vi "DownsampleStage3_5761_10MHzPID.vi"(8 "valid in":bool, 9 "reset":bool, 11 "Data in":fxp<+/-,32,14>[](array[numeric])=[0.0, 0.0, 0.0, 0.0, 0.0, 0.0, 0.0, 0.0]) -> (0 "valid out":bool, 3 "data out":fxp<+/-,32,14>[](array[numeric]))   [LabVIEW 2018]
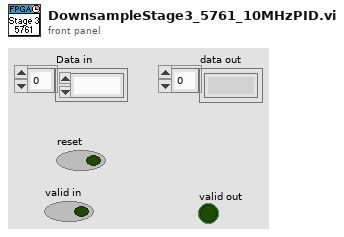
[diagram p1: front panel]
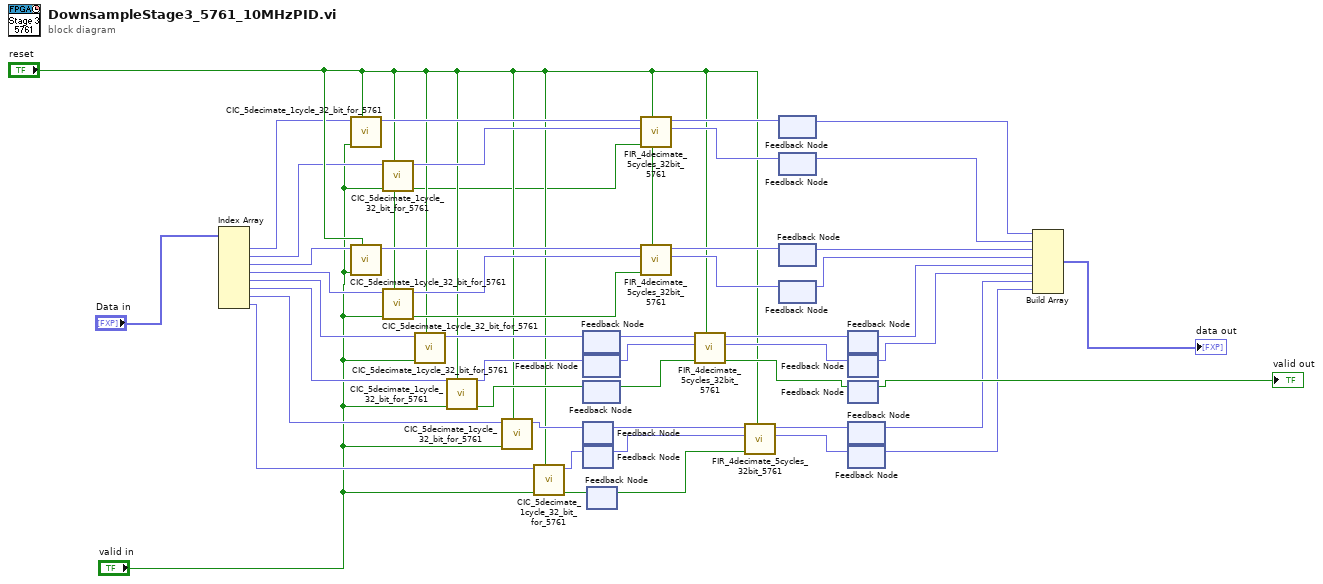
[diagram p0: block diagram]
diagram:
  n1 = Index Array(array="Data in") -> (element #1=w6:fxp<+/-,32,14>, element #2=w5:fxp<+/-,32,14>, element #3=w46:fxp<+/-,32,14>, element #4=w44:fxp<+/-,32,14>, element #5=w43:fxp<+/-,32,14>, element #6=w42:fxp<+/-,32,14>, element #7=w23:fxp<+/-,32,14>, element #8=w22:fxp<+/-,32,14>)  [unwired: 8 in]
  n2 = call "CIC_5decimate_1cycle_32_bit_for_5761.vi"("reset"="reset", "valid in"="valid in", "Data in"=w6) -> ("Data out"=w8:fxp<+/-,32,14>)  [unwired: 7 in, 1 out]
  n3 = call "CIC_5decimate_1cycle_32_bit_for_5761.vi"("reset"="reset", "valid in"="valid in", "Data in"=w46) -> ("Data out"=w35:fxp<+/-,32,14>)  [unwired: 7 in, 1 out]
  n4 = call "CIC_5decimate_1cycle_32_bit_for_5761.vi"("reset"="reset", "valid in"="valid in", "Data in"=w5) -> ("valid out"=w4:bool, "Data out"=w9:fxp<+/-,32,14>)  [unwired: 7 in]
  n5 = call "CIC_5decimate_1cycle_32_bit_for_5761.vi"("reset"="reset", "valid in"="valid in", "Data in"=w44) -> ("valid out"=w33:bool, "Data out"=w34:fxp<+/-,32,14>)  [unwired: 7 in]
  n6 = call "CIC_5decimate_1cycle_32_bit_for_5761.vi"("reset"="reset", "valid in"="valid in", "Data in"=w43) -> ("Data out"=w41:fxp<+/-,32,14>)  [unwired: 7 in, 1 out]
  n7 = call "CIC_5decimate_1cycle_32_bit_for_5761.vi"("reset"="reset", "valid in"="valid in", "Data in"=w42) -> ("valid out"=w39:bool, "Data out"=w40:fxp<+/-,32,14>)  [unwired: 7 in]
  n8 = call "CIC_5decimate_1cycle_32_bit_for_5761.vi"("reset"="reset", "valid in"="valid in", "Data in"=w23) -> ("Data out"=w17:fxp<+/-,32,14>)  [unwired: 7 in, 1 out]
  n9 = call "CIC_5decimate_1cycle_32_bit_for_5761.vi"("reset"="reset", "valid in"="valid in", "Data in"=w22) -> ("valid out"=w13:bool, "Data out"=w16:fxp<+/-,32,14>)  [unwired: 7 in]
  n10 = feedback #1() -> (w38:fxp<+/-,32,14>)  [unwired: 1 in]
  n11 = feedback-in #1(w41) -> ()
  n12 = feedback #2() -> (w37:fxp<+/-,32,14>)  [unwired: 1 in]
  n13 = feedback-in #2(w40) -> ()
  n14 = feedback #3() -> (w36:bool)  [unwired: 1 in]
  n15 = feedback-in #3(w39) -> ()
  n16 = feedback #4() -> (w18:fxp<+/-,32,14>)  [unwired: 1 in]
  n17 = feedback-in #4(w17) -> ()
  n18 = feedback #5() -> (w19:fxp<+/-,32,14>)  [unwired: 1 in]
  n19 = feedback-in #5(w16) -> ()
  n20 = feedback #6() -> (w12:bool)  [unwired: 1 in]
  n21 = feedback-in #6(w13) -> ()
  n22 = call "FIR_4decimate_5cycles_32bit_5761.vi"("reset"="reset", "valid in"=w4, "Q in"=w9, "I in"=w8) -> ("Q out"=w11:fxp<+/-,32,14>, "I out"=w10:fxp<+/-,32,14>)  [unwired: 4 in, 2 out]
  n23 = call "FIR_4decimate_5cycles_32bit_5761.vi"("reset"="reset", "valid in"=w33, "Q in"=w34, "I in"=w35) -> ("Q out"=w31:fxp<+/-,32,14>, "I out"=w32:fxp<+/-,32,14>)  [unwired: 4 in, 2 out]
  n24 = call "FIR_4decimate_5cycles_32bit_5761.vi"("reset"="reset", "valid in"=w36, "Q in"=w37, "I in"=w38) -> ("valid out"=w26:bool, "Q out"=w27:fxp<+/-,32,14>, "I out"=w28:fxp<+/-,32,14>)  [unwired: 4 in, 1 out]
  n25 = call "FIR_4decimate_5cycles_32bit_5761.vi"("reset"="reset", "valid in"=w12, "Q in"=w19, "I in"=w18) -> ("Q out"=w21:fxp<+/-,32,14>, "I out"=w20:fxp<+/-,32,14>)  [unwired: 4 in, 2 out]
  n26 = feedback #7() -> (w3:fxp<+/-,32,14>)  [unwired: 1 in]
  n27 = feedback-in #7(w10) -> ()
  n28 = feedback #8() -> (w2:fxp<+/-,32,14>)  [unwired: 1 in]
  n29 = feedback-in #8(w11) -> ()
  n30 = feedback #9() -> (w30:fxp<+/-,32,14>)  [unwired: 1 in]
  n31 = feedback-in #9(w32) -> ()
  n32 = feedback #10() -> (w29:fxp<+/-,32,14>)  [unwired: 1 in]
  n33 = feedback-in #10(w31) -> ()
  n34 = feedback #11() -> (w24:fxp<+/-,32,14>)  [unwired: 1 in]
  n35 = feedback-in #11(w28) -> ()
  n36 = feedback #12() -> (w25:fxp<+/-,32,14>)  [unwired: 1 in]
  n37 = feedback-in #12(w27) -> ()
  n38 = feedback #13() -> (→"valid out":bool)  [unwired: 1 in]
  n39 = feedback-in #13(w26) -> ()
  n40 = feedback #14() -> (w15:fxp<+/-,32,14>)  [unwired: 1 in]
  n41 = feedback-in #14(w20) -> ()
  n42 = feedback #15() -> (w14:fxp<+/-,32,14>)  [unwired: 1 in]
  n43 = feedback-in #15(w21) -> ()
  n44 = Build Array(w3, w2, w30, w29, w24, w25, w15, w14) -> (→"data out":fxp<+/-,32,14>[])
